vi "Set Processes Error Handler.vi"(8 "error in (no error)":errorcluster, 11 "Application In":refnum<class "Application.lvclass">) -> (0 "error out":errorcluster, 3 "Application Out":refnum<class "Application.lvclass">)   [LabVIEW 2020, in "Application.lvclass"]
uses:
  Application.lvclass
  C:/Git/astemes-triarc-framework/source/Framework/Error Handler Interface/Error Handler Interface.lvclass
  Application.lvclass/Application.ctl
  Process/Process.lvclass/Process.ctl
  Process/Protected/Messaging/Send Message.vi
  Process/Public/Lifecycle/Get Lifecycle State.vi
  Process/Private/SubVIs/Handle Debug Data.vi
  <vilib>/Utility/error.llb/Clear Errors.vi
  Logging/Log Debug.vi
  <vilib>/AdvancedString/1D String Array to Delimited String.vi
  <vilib>/Utility/High Resolution Relative Seconds.vi
  <vilib>/Utility/error.llb/Error Cluster From Error Code.vi
  Process/Public/Read Name.vi
  Process/Process.lvclass
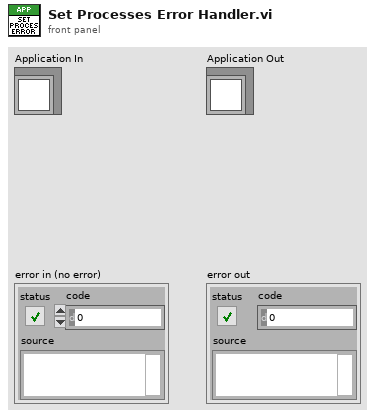
[diagram p1: front panel]
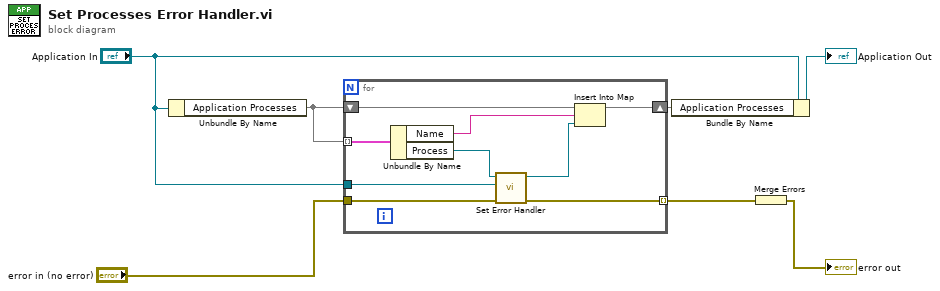
[diagram p0: block diagram]
diagram:
  n1 = Unbundle By Name("Application In") -> ("Application Processes"=w3:map{string, refnum<class "Process.lvclass">})
  n2 = for {
    tunnel: "error in (no error)" -> [w16]
    tunnel: "Application In" -> [w15]
    tunnel: [w14] -> w5 mode=indexing
    tunnel: w3 -> [w13] mode=indexing
    shift-right: [w8] -> w2
    shift-left: w3 -> [w11]
    n3 = Unbundle By Name(w13) -> ("Name"=w10:string, "Process"=w12:refnum<class "Process.lvclass">)
    n4 = call "Set Error Handler.vi"("error in (no error)"=w16, "Error Handler"=w15, "Process In"=w12) -> ("error out"=w14:errorcluster, "Process Out"=w9:refnum<class "Process.lvclass">)  [unwired: 7 in]
    n5 = Insert Into Map(map in=w11, key=w10, value=w9) -> (map out=w8:map{string, refnum<class "Process.lvclass">})  [unwired: 2 out]
  }
  n6 = Bundle By Name(cluster="Application In", "Application Processes"=w2) -> (→"Application Out":refnum<class "Application.lvclass">)
  n7 = Merge Errors(w5) -> (→"error out":errorcluster)
